vi "adam-5000-build-DO-cmd.vi"(8 "Output State":bool, 9 "DO Number":u8, 10 "Chassis Slot":u8=3, 11 "ADAM-5000: Chassis ID":u8=1) -> (3 "Command Out":string)   [LabVIEW 2020]
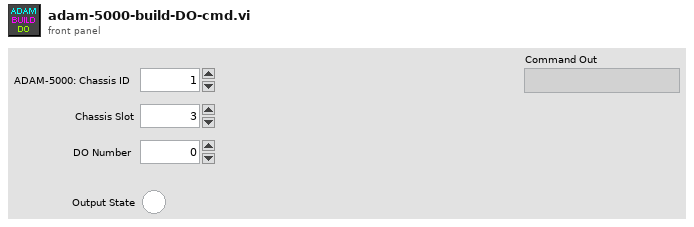
[diagram p1: front panel]
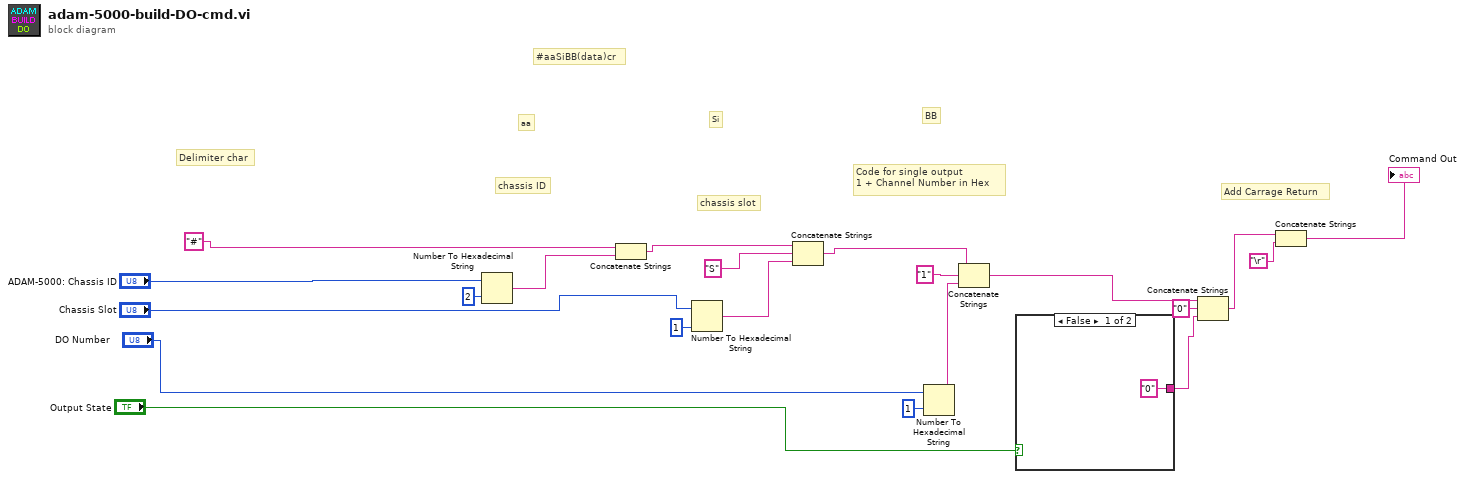
[diagram p0: block diagram]
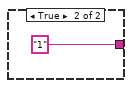
[diagram p2: hidden frame]
diagram:
  # "BB"
  # "Si"
  # "aa"
  # "#aaSiBB(data)cr"
  # "Code for single output\n1 + Channel Number in Hex"
  # "Add Carrage Return"
  # "chassis slot"
  # "chassis ID"
  # "Delimiter char"
  n1 = Number To Hexadecimal String(1:i16 2 ("width (-)"), 2:"ADAM-5000: Chassis ID") -> (0:w13:string)
  n2 = Concatenate Strings("#" ("string"), w13) -> (w17:string)
  n3 = Number To Hexadecimal String(1:i16 1 ("width (-)"), 2:"Chassis Slot") -> (0:w19:string)
  n4 = Concatenate Strings(w17, "S" ("string"), w19) -> (w12:string)
  n5 = Number To Hexadecimal String(1:i16 1 ("width (-)"), 2:"DO Number") -> (0:w6:string)
  n6 = Concatenate Strings(w12, "1" ("string"), w6) -> (w4:string)
  n7 = case shown="False" "Output State" {
    tunnel: ["0" ("string") "1" ("string")] -> w1
    frame False {
    }
    frame True {
    }
  }
  n8 = Concatenate Strings(w4, "0" ("string"), w1) -> (w5:string)
  n9 = Concatenate Strings(w5, "\r") -> (→"Command Out":string)
